vi "Read Recur Time.vi"(8 "error in (no error)":errorcluster, 11 "Weekly in":refnum<class "Weekly.lvclass">) -> (0 "error out":errorcluster, 2 "Recur Time":timestamp, 3 "Weekly out":refnum<class "Weekly.lvclass">)   [LabVIEW 2020, in "Weekly.lvclass"]
uses:
  Weekly.lvclass
  Weekly.lvclass/Weekly.ctl
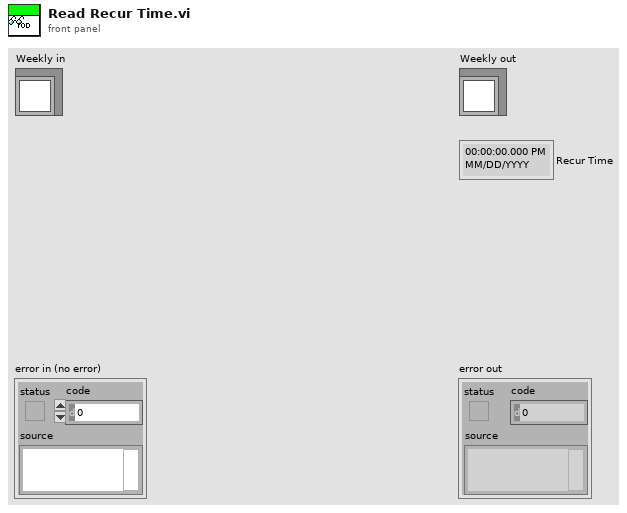
[diagram p1: front panel]
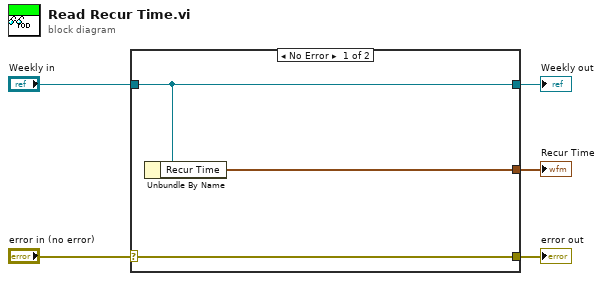
[diagram p0: block diagram]
diagram:
  n1 = case shown="No Error" "error in (no error)" {
    selector: "error in (no error)" -> [w8 w9]
    tunnel: [w8 w9] -> w4
    tunnel: [w7 w10] -> w2
    tunnel: "Weekly in" -> [w7 w10]
    tunnel: [w6 _] -> w1
    frame No Error {
      n2 = Unbundle By Name(w7) -> ("Recur Time"=w6:timestamp)
    }
    frame Error {
    }
  }
  "error out" <- w4
  "Weekly out" <- w2
  "Recur Time" <- w1
